vi "Day 9 Puzzle 2.vi"(11 "Path":path) -> ()   [LabVIEW 2021]
uses:
  SubVIs/Positions.ctl
  <vilib>/Utility/file.llb/Read Delimited Spreadsheet (string).vi
  <userlib>/_OpenG.lib/array/array.llb/Remove Duplicates from 1D Array (Variant)__ogtk.vi
  <userlib>/_OpenG.lib/array/array.llb/Remove Duplicates from 1D Array (String)__ogtk.vi
panel:
  out "Array 3":i32[](array[numeric])
  out "sum":i32
  out "size(s) 4":i32
  out "size(s) 3":i32
  out "Numeric":i32
  out "size(s) 2":i32[](array[numeric])
  out "Output Array 2":variant[](array[variant])
  out "Array 2":T1[](array[typedef])
  out "Output Array":string[](array[string])
  out "size(s)":i32
  out "element":string
  out "String":string
  out "match + rest of string":string
  out "Array":T1[](array[typedef])
  out "list of movements":string[][](array[string])
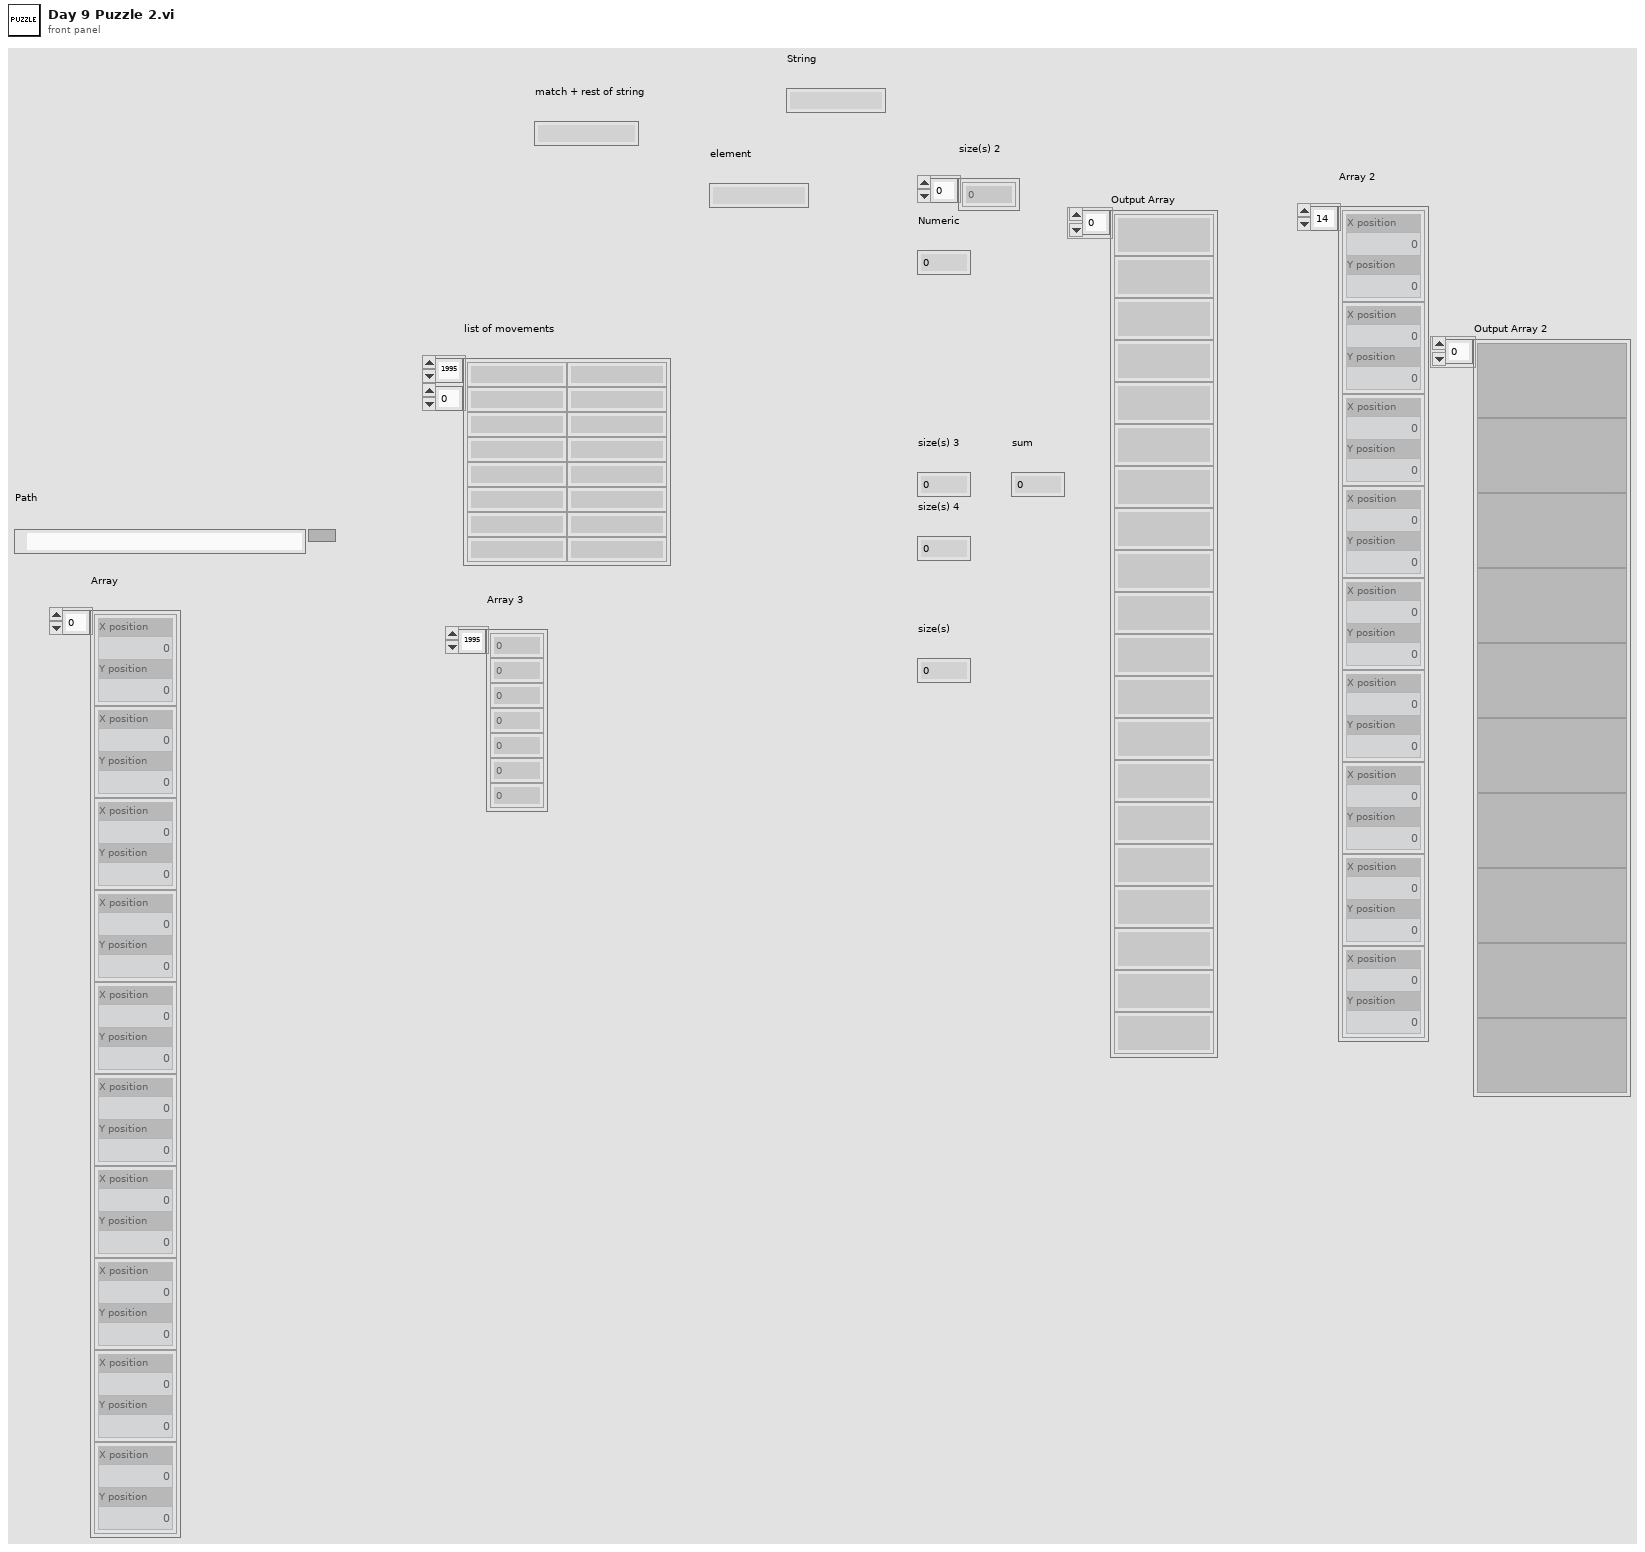
[diagram p1: front panel]
types:
  T1 = typedef "Positions.ctl" = cluster{"X position":i32, "Y position":i32}
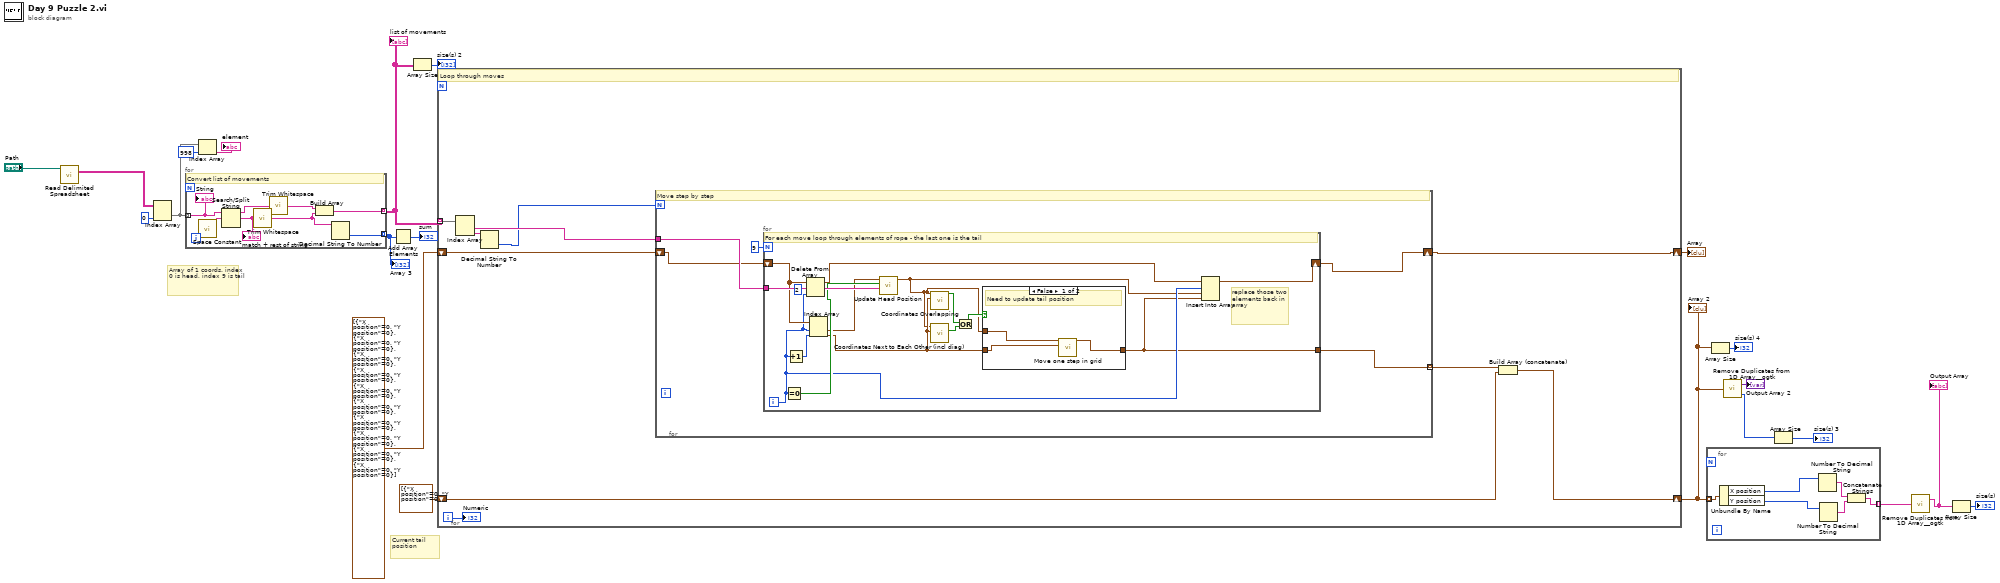
[diagram p0: block diagram]
diagram:
  # "Current tail position"
  # "Array of 1 coords. index 0 is head, index 9 is tail"
  n1 = call-poly <vilib>:"Read Delimited Spreadsheet.vi"("file path (dialog if empty)"="Path") -> ("all rows"=w17:string[][])  [unwired: 9 in, 5 out]
  n2 = Index Array(array=w17, index (col)=0 ("disabled index (col)")) -> (element=w15:string[])  [unwired: 1 in]
  n3 = for {
    tunnel: w15 -> [w29] mode=indexing
    tunnel: [w25] -> w8 mode=indexing
    tunnel: [w23] -> w2 mode=indexing
    # "Convert list of movements"
    n4 = call <vilib>:"Space Constant.vi"() -> ("String"=w28:string)
    n5 = Search/Split String(string=w29, search string/char (-)=w28) -> (substring before match=w26:string, match + rest of string=w27:string)  [unwired: 1 in, 1 out]
    "match + rest of string" <- w27
    n6 = call <vilib>:"Trim Whitespace.vi"("string"=w27) -> ("trimmed string"=w24:string)  [unwired: 1 in]
    n7 = call <vilib>:"Trim Whitespace.vi"("string"=w26) -> ("trimmed string"=w22:string)  [unwired: 1 in]
    n8 = Build Array(w22, w24) -> (w25:string[])
    n9 = Decimal String To Number(string=w24) -> (number=w23:i32)  [unwired: 2 in, 1 out]
    "String" <- w29
  }
  "list of movements" <- w8
  "Array 3" <- w2
  n10 = Index Array(array=w15, index=998) -> (element=→"element":string)
  n11 = Add Array Elements(numeric array=w2) -> (sum=→"sum":i32)
  n12 = Array Size(array=w8) -> (size(s)=→"size(s) 2":i32[])
  n13 = for {
    tunnel: w8 -> [w39] mode=indexing
    shift-right: [w30] -> w19
    shift-left: T1[] [{"X position"=0, "Y position"=0}, {"X position"=0, "Y position"=0}, {"X position"=0, "Y position"=0}, {"X position"=0, "Y position"=0}, {"X position"=0, "Y position"=0}, {"X position"=0, "Y position"=0}, {"X position"=0, "Y position"=0}, {"X position"=0, "Y position"=0}, {"X position"=0, "Y position"=0}, {"X position"=0, "Y position"=0}] -> [w31]
    shift-right: [w33] -> w4
    shift-left: T1[] [{"X position"=0, "Y position"=0}] -> [w34]
    i -> [w36]
    # "Loop through moves"
    n14 = Index Array(array=w39) -> (element #1=w38:string, element #2=w37:string)  [unwired: 2 in]
    n15 = Decimal String To Number(string=w37) -> (number=w35:i32)  [unwired: 2 in, 1 out]
    n16 = for {
      N: w35 -> [_]
      tunnel: [w42] -> w32 mode=indexing
      tunnel: w38 -> [w44]
      shift-right: [w40] -> w30
      shift-left: w31 -> [w41]
      # "Move step by step"
      n17 = for {
        N: 9 -> [_]
        tunnel: w44 -> [w56]
        tunnel: [w45] -> w42
        shift-right: [w47] -> w40
        shift-left: w41 -> [w53]
        i -> [w49]
        # "replace those two\nelements back in array"
        # "For each move loop through elements of rope - the last one is the tail"
        n18 = Equal To 0?(x=w49) -> (x = 0?=w52:bool)
        n19 = Increment(x=w49) -> (x+1=w55:i32)
        n20 = Delete From Array(array=w53, length=2, index=w49) -> (array with subset deleted=w48:T1[])  [unwired: 1 out]
        n21 = Index Array(array=w53, index #1=w49, index #2=w55) -> (element #1=w50:T1, element #2=w51:T1)
        n22 = call "Update Head Position.vi"("Direction"=w56, "Update?"=w52, "Head Position in"=w50) -> ("Head Position out"=w46:T1)  [unwired: 8 in]
        n23 = call "Coordinates Overlapping.vi"("Tail Positions"=w51, "Head Position"=w46) -> ("Checkbox"=w59:bool)  [unwired: 9 in]
        n24 = call "Coordinates Next to Each Other (incl diag).vi"("Tail Positions"=w51, "Head Position"=w46) -> ("Neighbouring"=w58:bool)  [unwired: 8 in, 1 out]
        n25 = Or(x=w59, y=w58) -> (x .or. y?=w57:bool)
        n26 = case shown="False" w57 {
          tunnel: w51 -> [w61 w63]
          tunnel: [w60 w63] -> w45
          tunnel: w46 -> [w62 _]
          frame False {
            # "Need to update tail position"
            n27 = call "Move one step in grid.vi"("Tail Positions"=w61, "Head Position"=w62) -> ("New Tail Position"=w60:T1)  [unwired: 9 in]
          }
          frame True {
            # "All good"
          }
        }
        n28 = Insert Into Array(array=w48, index=w49, new element #1=w46, new element #2=w45) -> (w47:T1[])
      }
    }
    n29 = Build Array (concatenate)(w32, w34) -> (w33:T1[])
    "Numeric" <- w36
  }
  "Array" <- w19
  "Array 2" <- w4
  n30 = for {
    tunnel: w4 -> [w69] mode=indexing
    tunnel: [w64] -> w12 mode=indexing
    n31 = Unbundle By Name(w69) -> ("X position"=w68:i32, "Y position"=w67:i32)
    n32 = Number To Decimal String(number=w68) -> (decimal integer string=w65:string)  [unwired: 1 in]
    n33 = Number To Decimal String(number=w67) -> (decimal integer string=w66:string)  [unwired: 1 in]
    n34 = Concatenate Strings(w65, w66) -> (w64:string)
  }
  n35 = Array Size(array=w4) -> (size(s)=→"size(s) 4":i32)
  n36 = call-poly <userlib>:"Remove Duplicates from 1D Array__ogtk.vi"("Input Array"=w4) -> ("Output Array"=→"Output Array 2":variant[], "indices of removed elements"=w6:i32[])
  n37 = Array Size(array=w6) -> (size(s)=→"size(s) 3":i32)
  n38 = call-poly <userlib>:"Remove Duplicates from 1D Array__ogtk.vi"("Input Array"=w12) -> ("Output Array"=w11:string[])  [unwired: 1 out]
  "Output Array" <- w11
  n39 = Array Size(array=w11) -> (size(s)=→"size(s)":i32)
